vi "Write MenuRef.vi"(8 "error in (no error)":errorcluster, 10 "MenuRef":refnum<k9>, 11 "Selector in":refnum<class "Selector.lvclass">) -> (0 "error out":errorcluster, 3 "Selector out":refnum<class "Selector.lvclass">)   [LabVIEW 2019, in "Selector.lvclass"]
uses:
  Selector.lvclass
  Selector.lvclass/Selector.ctl
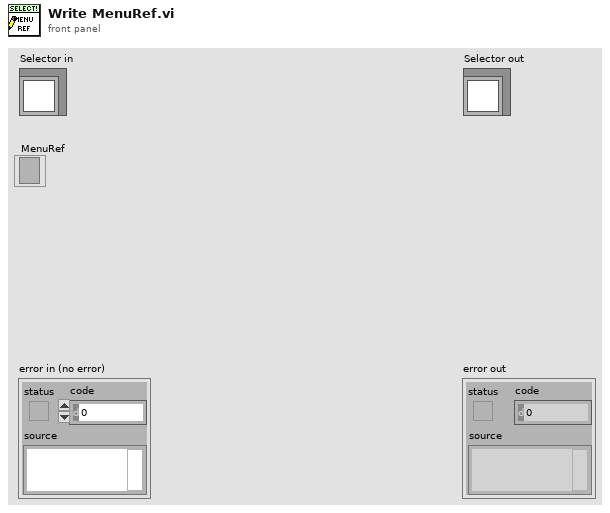
[diagram p1: front panel]
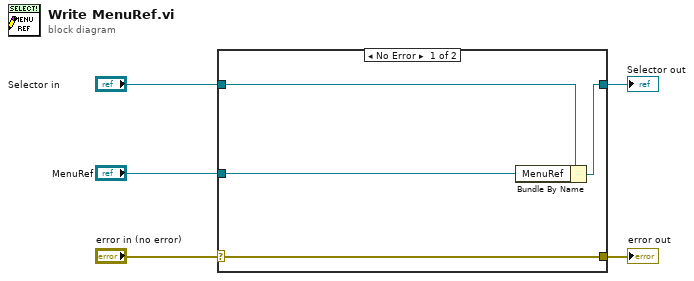
[diagram p0: block diagram]
diagram:
  n1 = case shown="No Error" "error in (no error)" {
    selector: "error in (no error)" -> [w9 w10]
    tunnel: [w9 w10] -> w4
    tunnel: [w7 w11] -> w2
    tunnel: "Selector in" -> [w8 w11]
    tunnel: "MenuRef" -> [w6 _]
    frame No Error {
      n2 = Bundle By Name(cluster=w8, "MenuRef"=w6) -> (w7:refnum<class "Selector.lvclass">)
    }
    frame Error {
    }
  }
  "error out" <- w4
  "Selector out" <- w2
